vi "Validate Library.vi"(9 "path in":path, 11 "Filename":string) -> (1 "path (dup)":path, 2 "valid":bool, 3 "Discovered Plugin":T1)   [LabVIEW 2021, in "CIFPluginLoader.lvclass"]
uses:
  CIFPluginLoader.lvclass
  CIFPluginManager/typedef/Discovered Plugin.ctl
  <vilib>/CIF Foundation/CIF Core/CIFCore/Common/Typedef/Version.ctl
  CIFPluginManager/typedef/Plugin Metadata.ctl
  CIFPluginManager/typedef/Loader Type.ctl
  <vilib>/Utility/LVLibp/NI_PackedLibraryUtility.lvlib
  <vilib>/CIF Foundation/CIF Core/CIFCore/Common/CIFCoreCommon.lvlib
  CIFPluginManager/CIFPluginManager.lvclass
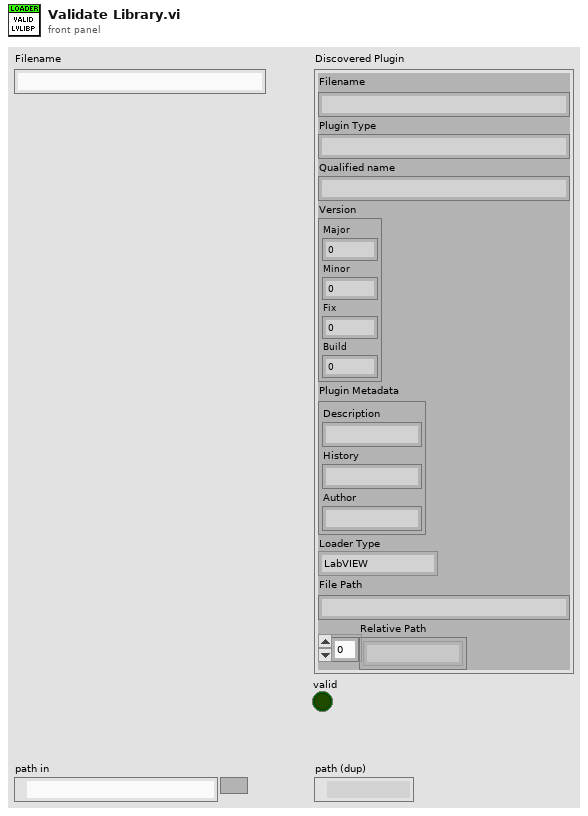
[diagram p1: front panel]
types:
  T1 = typedef "CIFPluginManager.lvclass/Discovered Plugin.ctl" = cluster{"Filename":string, "Plugin Type":string, "Qualified name":string, "Version":T2, "Plugin Metadata":T3, "Loader Type":T4, "File Path":string, "Relative Path":string[]}
  T2 = typedef "CIFCoreCommon.lvlib/Version.ctl" = cluster{"Major":i32, "Minor":i32, "Fix":i32, "Build":i32}
  T3 = typedef "CIFPluginManager.lvclass/Plugin Metadata.ctl" = cluster{"Description":string, "History":string, "Author":string}
  T4 = typedef "CIFPluginManager.lvclass/Loader Type.ctl" = enum16{"LabVIEW"}
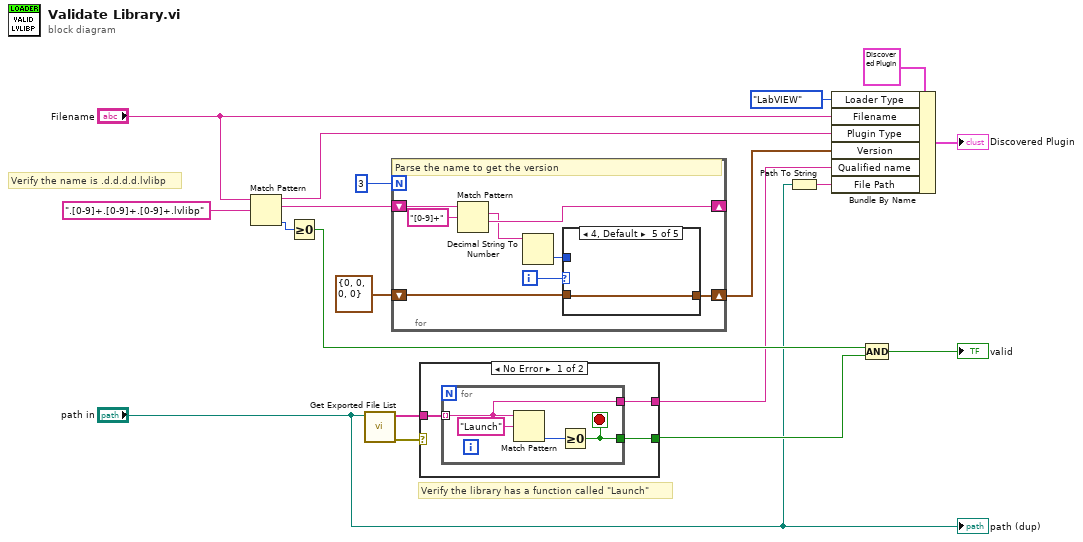
[diagram p0: block diagram]
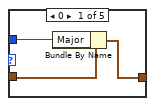
[diagram p2: hidden frame]
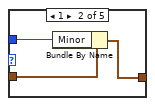
[diagram p3: hidden frame]
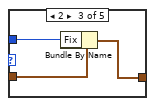
[diagram p4: hidden frame]
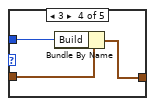
[diagram p5: hidden frame]
diagram:
  # "Verify the name is .d.d.d.d.lvlibp"
  # "Verify the library has a function called \"Launch\""
  n1 = Match Pattern(string="Filename", regular expression=".[0-9]+.[0-9]+.[0-9]+.lvlibp" ("Expression")) -> (before substring=w7:string, match substring=w16:string, offset past match=w12:i32)  [unwired: 1 in, 1 out]
  n2 = Greater Or Equal To 0?(x=w12) -> (x >= 0?=w10:bool)
  n3 = call <vilib>:"Get Exported File List.vi"("packed library path"="path in") -> ("error out"=w19:errorcluster, "qualified names"=w18:string[])  [unwired: 8 in, 1 out]
  n4 = for {
    N: 3 -> [_]
    shift-right: [w25] -> _
    shift-left: w16 -> [w27]
    shift-right: [w20] -> w13
    shift-left: T2 {"Major"=0, "Minor"=0, "Fix"=0, "Build"=0} ("Version") -> [w23]
    i -> [w24]
    # "Parse the name to get the version"
    n5 = Match Pattern(string=w27, regular expression="[0-9]+") -> (match substring=w22:string, after substring=w25:string)  [unwired: 1 in, 2 out]
    n6 = Decimal String To Number(string=w22) -> (number=w21:i32)  [unwired: 2 in, 1 out]
    n7 = case shown="4, Default" w24 {
      tunnel: w23 -> [w30 w31 w34 w37 w40]
      tunnel: w21 -> [w29 w33 w36 w39 _]
      tunnel: [w28 w32 w35 w38 w40] -> w20
      frame 0 {
        n8 = Bundle By Name(cluster=w30, "Major"=w29) -> (w28:T2)
      }
      frame 1 {
        n9 = Bundle By Name(cluster=w31, "Minor"=w33) -> (w32:T2)
      }
      frame 2 {
        n10 = Bundle By Name(cluster=w34, "Fix"=w36) -> (w35:T2)
      }
      frame 3 {
        n11 = Bundle By Name(cluster=w37, "Build"=w39) -> (w38:T2)
      }
      frame 4, Default {
      }
    }
  }
  n12 = case shown="No Error" w19 {
    tunnel: w18 -> [w43 _]
    tunnel: [w42 _] -> w9
    tunnel: [w41 _] -> w6
    frame No Error {
      n13 = for {
        tunnel: w43 -> [w44] mode=indexing
        tunnel: [w45] -> w42
        tunnel: [w44] -> w41
        stop <- w45 stop-if-true
        n14 = Match Pattern(string=w44, regular expression="Launch") -> (offset past match=w46:i32)  [unwired: 1 in, 3 out]
        n15 = Greater Or Equal To 0?(x=w46) -> (x >= 0?=w45:bool)
      }
    }
    frame Error {
    }
  }
  n16 = Path To String(path="path in") -> (string=w3:string)
  n17 = Bundle By Name(cluster=T1 {"Filename"="", "Plugin Type"="", "Qualified name"="", "Version"={"Major"=0, "Minor"=0, "Fix"=0, "Build"=0}, "Plugin Metadata"={"Description"="", "History"="", "Author"=""}, "Loader Type"=enum."LabVIEW", "File Path"="", "Relative Path"=[]} ("Discovered Plugin"), "Loader Type"=Loader_Type."LabVIEW", "Filename"="Filename", "Plugin Type"=w7, "Version"=w13, "Qualified name"=w6, "File Path"=w3) -> (→"Discovered Plugin":T1)
  n18 = Compound Arithmetic op=AND(w10, w9) -> (→"valid":bool)
  "path (dup)" <- "path in"
